vi "Create Referenced Object.vi"(8 "error in (no error)":errorcluster, 10 "Object Name":string, 11 "CS++Factory in":refnum<class "CS++Factory.lvclass">) -> (0 "error out":errorcluster, 1 "Attributes found?":bool, 2 "CS++Base Reference":refnum<class "CS++Reference.lvclass">, 3 "CS++Factory out":refnum<class "CS++Factory.lvclass">, 4 "Created new?":bool)   [LabVIEW 2012, in "CS++BaseClasses.lvlib" / "CS++Factory.lvclass"]
doc: "Create an referenced object by name. Object name is a kind of reference to attribute initialization data."
uses:
  CS++Factory.lvclass
  Reference/CS++Reference.lvclass
  Base/CS++Base.lvclass
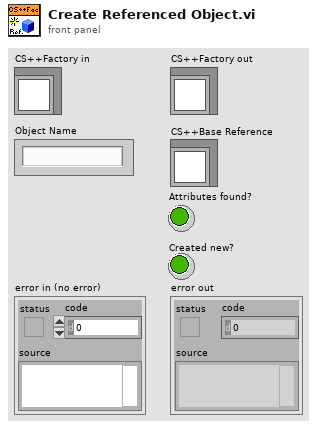
[diagram p1: front panel]
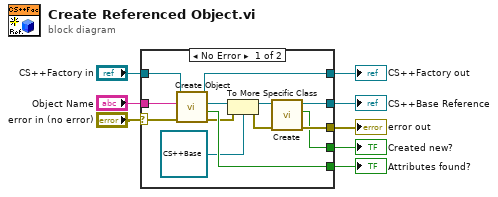
[diagram p0: block diagram]
diagram:
  n1 = case shown="No Error" "error in (no error)" {
    selector: "error in (no error)" -> [w9 w22]
    tunnel: "CS++Factory in" -> [w21 w23]
    tunnel: "Object Name" -> [w20 _]
    tunnel: [w19 w23] -> w6
    tunnel: [w18 _] -> w5
    tunnel: [w12 _] -> w4
    tunnel: [w11 w22] -> w3
    tunnel: [w10 _] -> w2
    frame No Error {
      n2 = call "Create Object.vi"("error in (no error)"=w9, "Object Name"=w20, "CS++Factory in"=w21) -> ("error out"=w17:errorcluster, "Attributes found?"=w18:bool, "LabVIEW Object"=w16:refnum<class>, "CS++Factory out"=w19:refnum<class "CS++Factory.lvclass">)  [unwired: 5 in]
      n3 = To More Specific Class(target class=refnum<class "CS++Base.lvclass"> refnum ("CS++BaseClasses.lvlib:CS++Base.lvclass"), reference=w16, error in=w17) -> (specific class reference=w14:refnum<class "CS++Base.lvclass">, error out=w13:errorcluster)
      n4 = call "Create.vi"("Error In"=w13, "Object"=w14) -> ("Error Out"=w11:errorcluster, "Created new?"=w10:bool, "Object Reference"=w12:refnum<class "CS++Reference.lvclass">)  [unwired: 7 in]
    }
    frame Error {
    }
  }
  "error out" <- w3
  "CS++Factory out" <- w6
  "CS++Base Reference" <- w4
  "Attributes found?" <- w5
  "Created new?" <- w2
